vi "Labview_with_sql.vi"() -> ()   [LabVIEW 2022 SP3]
panel:
  out "Data":string[][](array[string])
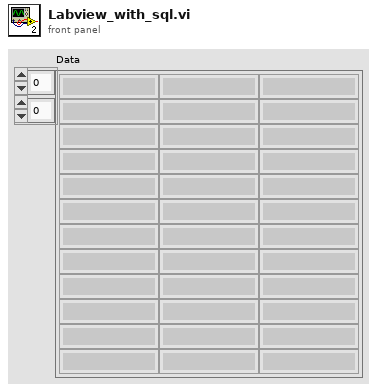
[diagram p1: front panel]
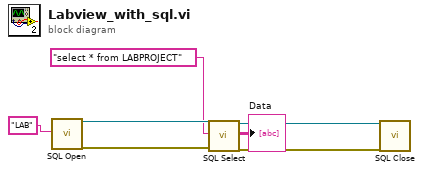
[diagram p0: block diagram]
diagram:
  n1 = call <vilib>:"SQL Open.vi"("ConnectionString In"="LAB") -> ("Connection Out"=w6:refnum<k7>, "Error out"=w5:errorcluster)  [unwired: 17 in]
  n2 = call <vilib>:"SQL Select.vi"("Connection In"=w6, "SQL Query"="select * from LABPROJECT", "Error in (no error)"=w5) -> ("Connection Out"=w4:refnum<k7>, "Data"=→"Data":string[][], "Error out"=w3:errorcluster)  [unwired: 14 in]
  n3 = call <vilib>:"SQL Close.vi"("Connection In"=w4, "Error in (no error)"=w3) -> ()  [unwired: 17 in, 1 out]
